vi "Configure Operation Mode Core.vi"(8 "error in (no error)":errorcluster, 9 "operation mode (Continuous)":i32(ring) items=["Continuous", "Burst"], 10 "channel name (\"CHANNEL1\")":string="CHANNEL1", 11 "CS++Fgen in":refnum<class "CS++Fgen.lvclass">) -> (0 "error out":errorcluster, 3 "CS++Fgen out":refnum<class "CS++Fgen.lvclass">)   [LabVIEW 2015, in "CS++Fgen.lvlib" / "CS++Fgen.lvclass"]
doc: "This VI configures the operation mode of the function generator. The operation mode determines how the function generator produces output on a channel. For example, you can select to generate output continuously or to generate a discrete number of waveform cycles based on a trigger event."
uses:
  CS++Fgen.lvclass
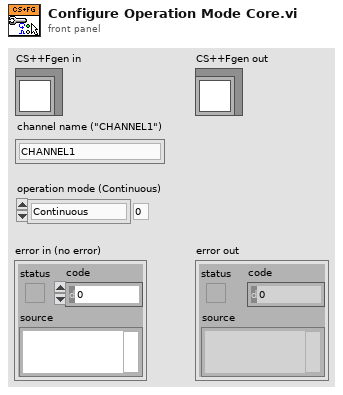
[diagram p1: front panel]
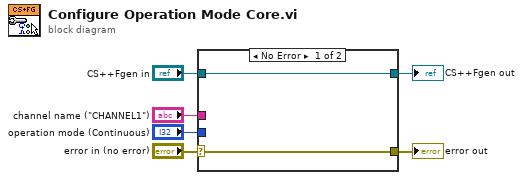
[diagram p0: block diagram]
diagram:
  n1 = case shown="No Error" "error in (no error)" {
    selector: "error in (no error)" -> [w7 w10]
    tunnel: [w7 w10] -> w5
    tunnel: [w8 w9] -> w3
    tunnel: "CS++Fgen in" -> [w8 w9]
    tunnel: "channel name (\"CHANNEL1\")" -> [_ _]
    tunnel: "operation mode (Continuous)" -> [_ _]
    frame No Error {
    }
    frame Error {
    }
  }
  "error out" <- w5
  "CS++Fgen out" <- w3
